vi "Main_04B.vi"() -> ()   [LabVIEW 2025]
uses:
  Utility/Universal Utility/TypeDefs_Utility/ENUM_8 Directions U-D-L-R.ctl
  Utility/Universal Utility/TypeDefs_Utility/Cluster_Row-Column.ctl
  b43e3300-6143-4e08-a70a-80936fe279ff.vi
  9e3f57c0-2ef8-4495-8287-c6a42a5fb955.vi
  <vilib>/Utility/error.llb/Trim Whitespace.vi
  <vilib>/Utility/error.llb/Trim Whitespace One-Sided.vi
  Utility/Universal Utility/TypeDefs_Utility/ENUM_4 Directions U-D-L-R.ctl
panel:
  out "sum":u32
  out "Array":bool[][](array[boolean])
  out "MATCH":bool
  in  "Select Data":enum32{"Example", "Puzzle"}(tab)
  in  "EX Target":u32=43
  in  "Example":string="..@@.@@@@.\n@@@.@.@.@@\n@@@@@.@.@@\n@.@@@@..@.\n@@.@@@@.@@\n.@@@@@@@.@\n.@.@.@.@@@\n@.@@@.@@@@\n.@@@@@@@@.\n@.@.@@@.@."
  in  "Puzzle":string="@@..@.@.@..@@.@@@@@.@@@@@@..@@.@@.@@..@@@.@@@.@.@@@@.@@@.@@@.@..@.@@@@..@@@.@@..@@@.@@@..@@@@..@.@@.@@@.@..@.@@@.@@@..@@@.@.@@@@@.@.@.@@@@@@\n@.@@@@@@....@..@@@.@..@.@.@@.@@.@@..@@@..@.@@..@..@@@.@@@.@..@.@.@@..@@.@..@@.@@@..@.@@.@.@..@@...@@@@@@@@.@@@.@@@.@@.@@@@@@@..@..@@@.@.@@.@\n.@.@@@@.@@.@@.@.@.@@.@..@@.@@..@@@@@@@@@@@@...@@.@...@@@@.@.@@.@@@.@.@@..@@.@@.@@.@@..@...@@@@.@@@@@@@@@@@.@@@....@@@@@.@.@...@@.@@@@@@@.@@@\n@@@..@@@@.@@@@@@@@.@@@@@.@@.@....@.@..@.@@@@@@@...@@@@@@@@.@@...@.@@.@@@@@@.@....@@.@@@.@.@@..@@@.@.@@@..@.@.@@@.@.@@@@@@@@...@.@@@@@@.@..@@\n@.@@@@@.@@.@.@.@.@..@@@@.@..@...@.@@@.@.@@@@.@@.@@@@@@.@@@@@..@@..@.@.@@.@.....@@@.@@@.@..@@@.@@.@..@@@@.@.@@@@..@@@@@@.@@@.@@.@@..@@.@.@@@@\n@@.@@@@@.@@@.@@@@@.@@.@.@@@@.@@...@.@@@..@@.@@.@@@..@@@...@@.@@@@..@@@@@@@...@.@@@@@@....@..@@@@@.@...@.@.@@.@...@@@@.@.@@@.@@.@.@@@@.@.@@@@\n...@.@@.@@.@.@.@@@@...@@@@@@@@@.@.@@@.@@.@@@.@@.@@@@.@@@@@@@@@.@@..@..@.@@@@@@@@@@@@...@.@.@@@.@.@.@.@@@.@..@@@@@@@@@@@.@@.@...@@@@@@@@.@@@@\n..@@@.@.@.@@@@@...@@..@@..@@.@...@@@.@.@.@.@.@@.@.@@@.@@.@.@@@@.@.@@@@@@@.@@.@.@@@@@@.@.@@@@@@@@@@@.@.@@@@@.@@@@@@@@@.@...@@@.@@@@.@..@@@@..\n.@@@@.@@@.@.@@@.@@@..@@..@@@@@@.@..@.@@.@.@@@@@..@@@@@@@@.@.@@@.@@@@@.@.@@@@...@@.@@@.@.@@@@@@.@@.@.@@@@.@.@@@.@.@@@@@.@@@@...@@@@@@@@@@.@..\n@.@....@@.@..@@@.@.@..@@@@.@.@@.@..@@.@.......@.@@@@@@@.@@@@@@@@.@@@.@.@@.@@@@.@..@.@@@@@@.@@@@....@@.@@@@.@..@@@.@@.@.@@@@@@@@.@@@@.@.@@..@\n@@@@@.@@.@.@.@@.@..@@@.@.@@@@.@@@.@.@.@@@.@.@@@.@@@@@..@@@@@@..@@@@@@@@@@@@@@.@@@@.@@@@...@.@@@@..@@@@@@@.@@@@.@@.@@@@@@.@@@.@.....@@@@@@.@.\n@.@@...@@@.@@..@@@@..@@.@@.@...@@@@@...@@@@.@@@.@@.@..@@@@..@.@@@@..@@@.@..@@@@..@.@@.@.@.@@....@.@@..@@.@@..@@@@...@@.@..@@@@@@@...@@@..@.@\n...@.@...@@@..@..@.@@@@.@.@....@@@@@@.@..@@@@@.@@@@@@@@@@.@@@@@@@@.@@..@@@@@@@@@@@@@@.@.@...@@....@@.@@.@@@.@@@@@@.@.@..@@@@@@.@.@.@@..@@@@.\n@@@@.@@@@.@.@@.@.@..@@@..@@@.@@@@@..@@@@@@.@...@.@@@.@.@..@@@@@@.@@.@@@.@@..@@@@@@@..@@@@@@@@..@@..@@@@@..@.@.@@@.@@..@.@.@@@@@@@.@.@@@.@@@.\n@@@@@@@@.@@@@@@@.@@@.@.@.@@.@..@@@@@@@.@@..@@..@.@..@.@@@@@@..@.@.@@.@.@@@.@.@@@@..@@@@@@@@....@.@.@@@@@@@@@.@@@..@@@@@@..@@@@...@@@...@.@.@\n..@@@..@.@@.@.@@...@@@..@.@@@...@..@@.@@@@@..@@@@.@@@@.@@@.@@.@@.@@@@@@@..@.@..@.@.@@@..@@@@@...@@..@....@......@.@.@.@.@@@.@.@@@@@@@.@@.@@.\n.@@.@@@@@.@..@@@@@@.@....@@@.......@..@@@.@@@...@..@@..@@@@..@.@@@@.@@.@@..@@.@.@@@@.@@.@@.@@@@@...@@@@.@@@..@.@.@@@.@.@@.@@@..@@@..@@@@@..@\n@.@.@..@.@.@.@@.@@@@@@@@@@@@.@@@@.@@..@.@.@@@..@@@@.@@@@@...@.@@.@@@@@@@...@@..@@@@..@@....@.@@@.@.@@@@@.@@@@@@@..@@@@@@@@@.@@@@..@@@.@....@\n@@..@@.@@.@.@..@@...@.@.@.@@....@@@@@@.@.@@@@@@.@..@@@@@@.@@@@..@.@.@.@.@.@@.@@...@@@.@.@@.@@.@@@@@@@.@..@@.@.@.@@..@.@@@@@@@@.@@@@..@@...@.\n.@@..@@@@@@@.@.@@@@.@@@@@@@@.@.@@@@@@@@@.@@@@@.@@@@..@@@@..@.@@@@.@.....@.@@.@@.@@@@@..@@@@@.@@@@@.@@@.@@.@@@..@@@..@@@@.@@.@@@@@@@@@@@@.@@@\n.@..@@@@@@@@@@@.@@.@@.@..@..@@@...@@..@@@.@@.@.@@.@.@..@@.@@.@@@@@.@@@.@.@@@@.@@@@@.@...@@.@@.@.@@..@@@.@@@@@.@@@@@.@....@@@@@@@@.@@.@@@@@@@\n@..@@..@@@@.@@.@.@.@.@.@@@@..@@.@..@.@@@@@@@.@@..@@@@@.@@@.@@@.@.@@.@@.@@@.@@@@@@@@@@@@@.@@@@@@.@@@@@@@...@@@@@@@.@@@@.@.@.@@@.@@@.@..@@@..@\n@@@@@@@@.@.@@..@.....@.@@@...@.@@..@@@..@..@..@@@.@@@@@@@@.....@..@@.@.@.@.@@@@.@@.@@.@@@@@@.@.@.@@.@@@@@.@.@@@...@@.@@@@@@@...@.@@.@@@..@.@\n.@@@@@@..@.@@...@@@@@@@@@@@.@@@@@..@...@.@.....@@@.@.@@@.@@...@.@.@.@@@@@@.@@@@@@.@@@@@...@@@@.@..@@.@@@.@@.@.@@@..@@@@@@@@.@@@.@@..@.@.@.@@\n@.@@.@@@.@.@.@.@@@@@@@@.@@@@..@.@@@@@.@@.@@....@..@@.@..@@@....@@..@@.@@@@@@@@@....@@.@@@.@@..@...@@@@@@@.@@@@@.@@@.@@@@@@@@@@...@@.@.@@@@@@\n@@@@@@@@@...@.@.@@@.@@.@@.@.@..@..@..@..@.@.@@@.@@@@@@@@@...@@@@@@@@@@.@@@.@@.@@...@@@@@@@.@.@@.@@@@@.@.@@..@..@....@.@@@.@...@..@..@@.@@@@@\n@@@@@@@@...@@@.@@@....@@@.@..@@@@.@@@@@..@@@...@@.@.@@@.@@.@.@@.@.@@@@.@@.@@@@@@@@@@@@..@@....@@.@@@@@.@@@@@....@@@....@@@@@.@.@@.@@..@@@@@@\n.@@@@.@@@@....@..@.@@@@@.@@@@@@..@..@@.@@@@.@@@..@@@...@.@@@.@.@@@@@@@..@..@...@@@.@@@.@@@..@@@@@...@...@..@@@@@.@@..@@...@@@.@@@@@.@@@...@@\n@..@@@...@@@.@.@@@@.@@@@@@.@@@@.@@.@@@@@@@..@@@..@@@@.@@@@..@@@..@.@@@...@@.@@@@..@@@@@@@@.@@@.@@...@@...@.@..@.@.@@.@.@@@@.@@.@..@@..@..@@.\n@@@@@@@..@@..@@.....@@..@@@..@@@@@..@@@@@.@@@@@.@..@@@@..@.@@@@...@..@@@.@.@@@..@@@..@@@@@..@@@@.@.@.@@.@@@@@@...@@@@@@@@@@..@@.@.@@.....@@@\n.@@@@......@@@.@@..@@@.@..@.@@@@@@.@.@..@@.@@@.@@@@....@@@@.@@.@@@@@@@.@.@@@..@@@.@@@@@@..@@@.@@@@.@@@@@.@@@@@@@.@@.@@@@@@.@@@@@@@@@.@..@@@@\n....@@@@@.@.@@@@@@@@@.......@.@@@@@@..@@.@@@@.@@@..@@@.@..@@@.@.@@.@@@.@@..@@@.@@@@@@@.@.@@@@@@...@@.@..@.@@.@.@@.@@@@@.@@@@@.@..@...@@@.@@@\n@@@@@@@@@@@@.@@.@@@.@@.@@.@@@..@@@@@.@@@.@..@.@.@@.@@.@@@@@..@@.@@..@....@..@...@@@@@..@..@.@.@@..@...@@@@..@.@@@@@@@@.@@@@@@@@@.@..@.@@@@@.\n@.@..@@@@..@@.@@.@.@@@@@..@@@@@@@....@@.@@..@@.@@@@...@@@@.@@@@@@@@@@.@.@@.@..@.@@@@@@@@.@@@..@@..@..@@@..@@@@....@@@@@@.@@..@@@@@@@@@@@@@@.\n.@@.@.@.@@@@@@.@@@.@@@@.@..@.@@.@@@@..@@@@@@.@@@.....@.@.@....@.@@@@@.@@@@.@@@@@@@@@@.@@@.@@@@@@@..@@..@@.@...@.@@@.@.@.@@.@.@@@@@@..@@@@.@@\n@.@@.@@@@@@@@@.@.@@.@@@@@@@.@@....@@.@@.@@@@@.@@@@.@...@@.@@@@.@@@@@.@..@@@@@@@.@@..@@@@@..@@.@...@@.@@.@@@@.@@@@..@..@@@@@.@@@.@@.@@@@@...@\n@.@@@.@.@..@.@@.@.....@.@.@@@@@@@@@.@@@@@@@@@@.@..@.@@.@@...@@@.@.@@.@.@.@@.@@@..@@@@@@.@@@@@@@@@.@....@.@@@@@@.@@@@@.@@.@.@@@@@@@.@@@@@@@.@\n@.@...@@@...@@.@@..@@..@.@.@@..@.@.@..@..@@@@@@@..@@@@@@@@@@.@@.@@@.@@@@..@..@.@@..@@@.@.@.@@@.@.@.@@@@@@....@.@@@@@@@@@.@@@@@@..@@@.@@@.@@@\n.@@@@.@@@.@.@.@@..@@@.@@@@..@@@.@@.@@@..@@@.@@..@.@@@@@@..@@@@@.@@@.@@..@.@.@@@@...@@.@...@.@@@.@@@@.@@@.@..@@@@..@@@..@@.@@.@.@@.@.@.@@.@@@\n..@@@@..@@@..@.@@@@@.@..@.@@.@...@@@@@@@@..@.@@@@@@...@@@@.@.@@@....@...@@.@..@@@@@.@.@.@.@@.@@@@@.@@@@@..@@@@@@@..@@.@@.@@..@...@@@@@@@.@.@\n.@@@@.@@@@.@@@@@..@..@@..@.@.@@....@@@@.@...@@@@@@@@..@.@..@.@@@@@@@@@@@.@.@@..@.@@.@.@@@@@@.@@@.@@@.@@@..@@..@@..@.@@...@@.@..@..@.@@@.@.@@\n.@@@@@@@@@@@@.@@@.@@...@..@..@..@.@.@@@.@..@.@@...@@.@@..@@@@@@..@@@@@@@.@.@@@@@.@@.@...@@.@@.@@@@@@.@@@.@.@@@@..@...@@@@...@@.@@@@@@@@.@@.@\n.@@@@.@..@..@.@@@@@.@.@@@@.@.@.@.@..@.@@@@..@@@..@@..@..@@@@@.@.@@@@...@..@....@..@@.@...@@.@.@@@.@@@@.@@@.@@@@@....@@@@.@@@.@..@@@@@@@..@.@\n@@@@@@@@.@@@...@@..@.@.@.@@.@@.@@..@@@..@@.@@@@@@.@@.@@...@.@@@@..@@@@@..@@..@.@@@@@@@@@..@@...@@.@@@.@@@@@@@.@@..@@.@@@@.@...@.@.@..@@.@.@@\n@.@@@.@.@@@@@@@@@@@..@@...@.@@@..@@@@@..@.@@@..@.@@@@.@@@@@@@@@.@.@@@.@@@@@@@..@.@@...@@@..@@.@.@@.....@@@.@@.@..@@.@..@@@.@.@.@.@@@.@@.@@@@\n@.@.@....@@@.@@..@@@.@@@@@@@.@.@@.@.@@@@@@@.@@.@@@@@.@.@@....@.@@@..@@@@@.@@@@.@.@@@.....@@@@@@@@@@..@..@@@@@@..@.@@@@@@@.@.@@.@@@.@@@@.@.@@\n.@@@@.@@@.@..@@@.@@@.@..@@.@@.@.@@.@@@.@.@@@@@.@@.@..@.@.@@@@.@@@.@@.@@@..@.@.@@@..@@@@@@@@@@@.@@@@@@@@@.@@@@@@..@@@...@@@.@@.@.@@@@@@.@@@@@\n@@.@.@@@@@@@@@..@@...@@@@..@@@.@@.@.@.@@....@@..@@.@@..@@@.@@.@..@@.@@@@.@@@@@@@@.@@@@@@@@@..@.....@@@@....@@@@@...@...@..@@@@@.@@.@....@.@@\n.@@.@@...@@@@@@.@@.@@@@.@.@@@@.@@.@..@@@@.@...@@@@.@.@....@.@@@@@@@@@.@@..@@.@.@@@@@@.@.@@.@.@@@@@@....@.@@@@@.@.@.@.@@@@..@@@@.@.@..@..@@@@\n.@@@@@.@@@.@.@@...@@..@@@..@@...@@@@..@...@.@...@@.@.@@@@...@@@..@@@@@@@@@.@@.@..@.@.@@.@@@.@@@..@@@@...@@@@@@@..@.@@@@@@.@@.@.@@@@.@...@@.@\n@@..@.@.@@.@.@@.@.@@@..@@...@@@@@@@@@@.@.@@@@@@.@.@.@@..@@@..@...@@@@..@......@.@.@..@.@.@.@.@@@@.....@.@.@.@@.@@.@.@@@@@@.@@@@@..@.@.@..@@@\n.@@@@@@@@@@.@@@@..@.@.@.@@@@@@@@.@@@.@@.@@..@@..@@@.@@..@.@.@.@@@..@.@.@@@.@..@@@.@@.@.@..@@@...@.@@@@...@@@.@.@@.....@@...@.@@.@@@@@.@@@@@.\n.@@@..@@@@@@@.@@@.@@@@..@@@..@..@@@..@@@..@@.@@.@@@@@@@.@.@@@.@.....@@@@@.@@.@@..@@@@.@@....@@@..@@@@.@@@@@@.@@.@..@@@.@..@@..@..@@.@@@.@@..\n@@@@@@..@.@@@@@.@@@@.@..@.@@@@@..@@@@..@..@@@@@.@@@@@@@.@..@@..@@@@@@@@..@@@@.@.@@.@@...@.......@@.@..@@@@.@..@@@@...@.@@@.@......@@...@@@..\n@.@.@.@....@.@.@@.@@@@@@@.@..@.@..@@.@.@.@@@@@@..@...@...@.@.@.@.@@@@@@@@@..@@@.@@@@@@@@@.@..@@@@@@.@@.@@@@@@.@@.@@...@@@@@@.@@@.@@.@..@..@@\n.@@@.@@@@@@@@.@@@.@..@@.@..@..@@.@@@..@@@@@@.@@@@..@@....@@@@.@.@@.@@.@@@..@@@@@@@....@..@@.@@@@@..@..@...@@.@@@@@.@@.@@@@.@@@@@@.@..@.@@@.@\n@..@...@@@@..@@..@@..@@@.@.@@@@.@..@@@.@.@.@@@@@.@@...@..@@...@....@.@.@@@@@.@@@.@@..@@.@@@.@.@@..@@@@..@@@@@@@@@.@@@@@.@@.@@.@.@@.@.@.@@@.@\n@.@.@@@.@..@.@.@.@.@@@@@@@.@.@@.@..@@@.@@@@@@@...@@@.@@@.@@@@.@@@....@@@@@@@.@@.@.@@...@..@@.@..@.@@.@.@@@@..@@@.@@@@@@..@@@..@.@@@@@@@@@@.@\n.@@.@@@@..@..@@.@.@.@@.@@@@..@@.@....@@@@.@@@.@@@.@@@@@@@@.@@.@@@.@@@@.@@@@@@@@@.@@@@..@@.@..@@@.@.@@@@@@@@@@@.@@.@.@.@...@@@@@.@@.@...@@@@@\n.@..@@...@@.@@@@@@@@@@.@@@.@@.@@@@@@@.@@.@@@@.@@..@@.@.@@.@@@.@@@@.@.@@@@..@...@.@...@@@.@@@@@..@@@@@@@..@.@@@.@.@.@.@.@@.@@@@..@.@..@.@.@@.\n.@..@...@.@@.@..@@@@@@..@.@@@@@@...@@..@@.@@@@.@....@.@@@..@@@@..@@.@.@..@.@@.@.@.@@@.@..@.@@@@@@.@@@.@@.@.@..@@.@@.@.@@@.@.@.@.@@@.@@@.@@..\n.@@@.@.@..@..@@@..@@@.@@.@.@@@.@@@.@@@.@@@..@@@@@@..@@@@@@@.@@@@.@.@...@@@@@@@.@@@@...@..@@@@.@.@@@......@@@.......@@.@..@@@@@..@.@.@@@...@@\n.@@@@@@.@@@.@@@@@@@.@@.@@.@@@@@..@.@.@.@..@@.@.@.@@@.@.@@@.@@@.@@.@@..@@@..@@@@...@@..@.@.@@@..@@..@.@@@.@..@.@@@@@@@@@...@@@@.@@@@@@@.@.@.@\n@.@.@@.@@@....@@@@@@@.@@@...@@@..@.@@@@@@@@@@@@.@.@@@@@.@@@.@@.....@.@@@....@.@@....@@@@@@@.@@@@@.@@@.@.@.@@.@@@@@@@@..@.@.....@@@@@..@@@@.@\n@....@...@.@.@..@@@@@......@.@...@.@.@..@@.@@@@@@..@@@@.@.@.@.@.@.@...@@@@.@@@.@...@...@@@...@@@@@@@@@@@..@@@..@.@@@@@@.@@@@@....@@@.@@.@..@\n@@@@.@..@@@.@@@..@@.@@@@@@.@.@.@.@@@@@@@.@.@@.@@@.@@...@@.@.@.@@..@@@.@@@@@.@@.@.@@@@@.@@@@@@.@@.@@@@@.@.@@.@@....@@....@....@@@@.@@.@@@..@@\n@.@@@@@@@@@..@@@@@..@.@@.@..@@@.@@@@@@@@..@@@@@..@@@.@.....@@@..@.@@@@@@..@@..@@@.@.@..@.@@.@@@@@@.@.@@.@@@.@@.@@.@..@.@.@@@@..@.@@@@..@.@.@\n@@@@@.@.@.@@...@@...@@@@@@@@.@..@..@@@@..@@@..@.@@.@.@@@.@.@@@...@.@@@..@@@@@@@@@....@@@@@.@@@.@@..@@...@@@.@.....@@..@@@@@@@@@..@@@@@.@@@@@\n@@@..@@@.@@@@@@@@@@@@..@..@.@@.@@@@@@@@@@@@@.@@@@@@.@..@.@@@@@@@.@@@@@.@@@@@@@...@@@@@...@@.@.@@@@..@@@@@@.@@@@@..@@@@@@.@...@..@@@.@@.@.@@.\n.@@..@@@@@.@@.@@@@@@.@@@.@@.@.@@@@.@@..@@@....@@@@@@@.@@....@@@@@@.@@.@@...@..@@@@@@..@.@.@@@@@@@@@@.@@@@.@@@@.@.@@@@...@.@.@@.@.@@.@.@@@@..\n@.@@.@@.@@@@@@@@@.@@@@@@@.@@@..@..@.@...@..@..@.@....@@.@@.@@@@.@.@@.@@.@@.@.@@@@@@@@@@@.@.@@@..@@@..@@@.@@@@@@@@.@.@@@@@@@.@@.@..@@@@@@@@@@\n..@@..@.@@@@@.@@@.@@@.@.@@@@.@.@@@@@@@@@@@@@.@@@@...@@@@@@@@@@.@.@@.@...@@@@@..@@.@@@@..@@@...@..@@@.@@@.@@@..@@@@.@.@@.@@@.@.@.@.@@@.@@.@..\n@@..@@@@@...@@@.@@@@.@...@@@@@@@.@@@.@...@@@@@@@..@..@@@@@.@.@@.@.@@.@.@.@@@@@@...@.@....@@@..@.@@@@@@@@@@@@.@..@@@@@@@@@.@@.@@@@@..@@@@.@@.\n@.@@.@@..@...@@@@@@..@.@@...@@.@@@@@@.@.@...@@.@@@.@.@@@@@.@@@@@.@.@@@.@.@@@@@@@@@.@@@.@.@@@@@@@@@@@@.@.@@@.@@.....@.@@@@@@@@@@@@@@@..@...@@\n@.@.@.@.@.@@...@@@@@@.....@.@.@..@..@@@@@@@..@@@@@@....@@.@..@@..@.@@..@@@.@@.@@.@@@@@.@....@@@@....@.@@@...@..@...@@.@@@@@@@@@@.@@...@@@@.@\n@@@.@@@...@@@.@@@@@@@@.@.@@...@@@@..@..@@@@@..@@@@@@@@@....@@@@@.@@@....@.@.@.@.@@.@@@@..@@@.@@..@.@.@@@@@@@@@@@@@@@@.@.@.@@@@@....@..@@.@@@\n...@@@.@@.@@.@@.@@...@.@.@...@@.@@.@@.@..@@@@.@@.@@@@.@@.@@..@@@@...@@@@@.@..@.@@@@@@..@@..@@@.@.@.@@..@@@@@@..@@..@.@@@@@@@@.@...@@.@@.@@.@\n@@@@..@@.@@..@.@@@@@.@.@@@@.@@..@..@@.@.@@@@..@@@@@@@@@@@@@.@.@@@@.@.@@@@@@.@...@@@@.@.@@...@.@@@@.@@@..@@@..@.@@@@@..@.@@.@@.@@@@@@@@.@@@@.\n@@@..@@..@@@@@.@@.@..@@@.@..@.@@.@@..@.@.@@.@....@@@...@@@.@@@..@.@.@.@@@.@.@.@....@@....@@@@@.@@@@@@@.....@@..@.@@@.@@@@....@@..@@@.@@.@.@.\n@@.@..@@@@@@@.@.@@.@@@.@@@.@@.@@@@@@@@@@.@@@..@.@@@@..@@.@@.@.@.@@@.@.@@@@@@......@@@..@@@.@.@@.@@@@..@@.@@.@.@@..@.....@@@@@.@.@@.@.@.@.@.@\n@@@.@@@@..@.@@.@@@.@.@@@.@....@.@.@@..@..@@.@@@@@@.@@.@@@@.@@@@@@@@@@@@@..@.@.@@..@..@@.@@@@.@@.@@.@@..@@@@@@.@@@@@.@@.@@@.@@.@...@@.@@.@.@@\n@.@@@@@@@..@.@@@.@.@@@.@.@@@@@..@@@@@...@@@@.@@..@@.@.@...@@@@@@@@@@@.@@@@@@...@@@@@.@@@@@..@@@.@@.@..@.@@@@.@@.@@@.@@@.@@@.@.@@@@@@@@@..@@.\n@.@@.@..@@.@@@@@.@@.@@@.@..@..@@@.@.@.@@@@@.@@..@.@@....@@@@@.@..@@.@@.@@.@@.@@.@.@@.@@@.@@@.@@.@.@@@.@@@@@@@..@@@.@.@@.@.@@.@@@.@@...@.@@@@\n@@......@@@@@.@.@.@.@@@@..@@.@@@@@@@@@.@@@@.@@@.@@@.....@@@@@@@@..@@@@.@@...@@@@@@@@..@.....@.@@@..@.@@@@@@@@@.....@@@@@@@@.....@@.@@..@@.@.\n@@@...@@.@.@.@@.@@.@..@.@@.@@@@@..@..@.@@@@@@@.@@.@@@..@..@.@@@@.@@.@@@@@@@@@@@.@..@@@@.@..@@@@@.@.@@@@@@@@@..@@.@@@@...@@@@@@@.@@..@@.@@@@@\n.@.@@@.@@@@.@@.@@@@@...@@..@@@@@@@@@.@.@@..@.@@.@@@.@@@@@@.@@@@...@@.@@@..@...@@.@@@@.@....@@@.@....@....@@@@@@.@@@..@@.@@..@@...@@@..@.@@@.\n.@....@.@@@@@@@@@@...@@@@.@.@.@.@@@.@@@@@@@@@.@@.@@@..@.@.@@@@.@...@@@@..@.@@@@..@@.@@@@.@@@@@@.@@.@.@@.@..@@@@@@@@@@@@@@@@.@@@@@@.@.@.@.@..\n..@@@.@..@@..@@@@@@@..@@@.@@@@..@@..@@@@.@@@@..@@@.@@@.@@@@..@@..@.@.@.@@@@@@@...@@.@@@@@@.@@.@@@.@@@.@@@@@@@@.@.@@@@@@@@@.@.@....@@.@@@@@@.\n@.@@@.@@@@@.@@@@@.@@@...@.@@.@@@@@@.@..@.@@@@@@.@@.@@@@@@.@@@@@.@@@@@@...@@..@@@@@..@.@@@.@.@@.@.@.@@.@@@@.@.@..@@@.@.@@@...@@@..@@.@@@@@..@\n@@@.@@@.@@..@..@@@....@.@@@..@....@.@.@@@.@....@@@..@@.@@@@.@.@@...@..@.@@@.@@@@@@@@@..@.@@...@@@.@@@@@...@@....@@@@@@.@....@@@.@@.@@..@@@@@\n@.@..@...@@..@.@@@..@@@@@@.@..@@@..@@@@@.@@@@@@@.@..@@@@...@@.@@@@.@@@@@.@.....@@@@@.@@@@@.....@@.@..@@.@@@@@.@@.@@@@@.@@.@@.@@.@.@@..@.@.@.\n@..@@@@@@.@@...@.@..@@@@.@@@.@@@@@@@@.@..@@@@...@@@@@@@.@.@@.@@@@..@....@.@....@...@@.@@.@.@.@.@.@@.@@.@@.@@@..@@@@.@@@@.@@@.@.@@...@..@@...\n@@@@@@.@@@@@.....@@@@@@@@@@@..@.@@@@@@@@..@...@.@@.@@@@.@@@.@@@.@.....@.@@@.@@..@@@@...@@..@.@@@@.@@.@@@@..@@.@..@@@@@@@.....@@.@...@@..@.@.\n@@@.@@@@..@@.@.@@@@..@.@@.@@..@@@..@@.@@.@@...@@@@@..@..@@@@.@@.@@@@@.@@@..@@.@@@@..@.@.@...@@.@@@@@@..@@@@@@@..@@@@@@@.@.@.@.@.@...@@@.@@.@\n@@@@.@..@@.@.@.@@@.@..@@.@@@@@@@..@@@@@@@@@@@.@@@@@@.@@.@.@@.@@..@@@.@@@@@.@@.@..@@@.@@@@.@@@....@@@@@@@.@....@.@@@@@@@.@@@@.@@@...@.@@.@@@@\n@@.@.@@...@@@.@@..@@.@@@@.@@.@@.@..@.@..@@@@@@..@...@@..@@@.@.@@@@.@@.@@@.@.@@.@.@@@@@...@.@.@@@..@@@@.@@@@@.@...@@@.@@@@.@@.@...@.@@@.@@@.@\n@.@.@..@@@@..@@.@.@..@@@@@.@@@.@....@@.@..@@.@.@..@@..@....@@@.@@@..@@.@@@@@@.@.@.@@@@@.@@..@.@@.@@@..@@@.@@.@@@@..@@@@@@@@@.@@@@@@.@@@@.@.@\n.@.@@.@@@.@..@@..@@..@@@.@.@@.@@.@@.@....@@.@@.@.@@@@@.@@@.@.@....@.@@@.@@@@@@@@@@.@@@..@@@@....@@.@@...@.@@...@.@@....@...@.@@.@.@@..@.@@@@\n.@@@@@@.@@@@@@@..@@@@@@@@@@..@..@@@@@@@@@@....@.@@@@@@.@@@@@@@@@.@@..@.@...@......@.@@@@@.@.@.@@.@@....@@..@@@..@@.@@.@..@@@.@@...@@@@@@@@@.\n@@@.@@@@@@.@...@.@@...@..@@@@.@@@@@..@.@@.@@@@@@@....@@@.@.@@.@..@.@.@@.@.@@..@.@@@@.@....@...@@@.@@@@.@@@@@@@@.@...@@@@@@@@@@.@@@..@.@..@@@\n@@@@.@@..@..@@@@.@.@@@..@@.@@@.@@.@@.@@@..@@@@.@@@@@@.@@..@.@@@.@.@@...@..@@@...@.@@.@@.@.@@@@.@.@...@@@.@@@.@@.@.@@.@@.@@@@@@.@@@@.@@..@@@@\n.@.@.@@@@@@@@@.@...@..@@.@@@@@@@@@.@@@@.@@..@@.@@.@@@@.@@@@@@@..@@..@...@@.@@@@@@@@@.@@@@@@@@@@@@....@.@@@.@.@@@..@@..@@.@@.@@.@..@@.@.@@@@@\n.@@.@@@....@@...@@.@@@.@@...@@..@@.@@..@@@@...@@@@@..@@.@..@.@@@.@.@..@..@@@@.@@..@@......@.@@@@@@.@....@.@.....@@@.@@.@@@@..@@.@@@@..@@..@@\n..@.@@@@@.@@.@..@..@@.@@@@.@@@...@..@@@.@..@@@.@@@.@@...@@@@@@.@@.@.@@@@..@@@@@.@@@.@.@@@@@...@...@@@@.@@@@@.@@@@@@.@@@.@@@@@@..@....@.@....\n......@.@@@@@@@..@@@..@@@@@.@@@.@@@.@@.@.@.@@..@@@@.@.@@...@.@@@@.@@.@.@.@@@@@.@@@@@@@...@@.@@@@@..@@@.@@@.@.@@@@...@@@@@@.@@@.@@@@.@..@@@.@\n@.@@@@.@@.@@.@.@@.@@@@@@@@@@@@@@@@@@@@@@.@@@@.@.@.@@@@.@..@@@..@.@..@@@@@..@@@@@.@..@@.@@@@@@.@@@@@@.@@.@@@@@.@@@.@@@@.@.@@@@@@..@@.@@..@@@@\n.@@@@.@@@@@@@@.@@@@@.@..@.@..@..@@.@@@@@...@@@.@@@@@@.@@@@@@@@.@.@@@@..@@..@@@.@@@@@@.@.@@@@@@@.@@@.@..@.@@.@.@..@@@.@@@@@.@@@@@...@@@.@@.@.\n@...@@@@..@@.@@@.@@@.@@@@@.@@@....@@@@@@@@@@.@@..@.@.@.@.@@..@.@@@@@.@@.@.@@@@@.@@@.......@..@@......@@..@@.@@@.@@@@@@.@.@@@@@.@@@@.@@@@..@.\n.@@....@..@.@.@@@@@@@@@@@@..@@@@.@@@@@@@@@..@@.@.@@@@.@@.@@@@@@@.@@@..@.@.@@@@.@.@@@@@@@@.@@@@..@@@..@@@.@@@.@@@@......@@.@@..@@.@@@@.@...@.\n@@@@@@@@@@@@@@@@@@.@@.@...@@.@..@@.....@@@@@@..@@.@.@@..@..@@@...@@....@@@@@.@@@@.@@.@@@@.@..@@.@@.@@@.@@@......@...@...@@@@@@@@@@@.@@@@@.@@\n@@...@@@.@@.@.@.....@.@@@@@@@.@.@.@@@..@@@@@..@@.@@@@@@@@@@@@@@@.@@..@@@@...@@@.@@.@@.@@@@@.@..@@@.@@@@@..@@....@.....@@@..@@@@@@@@....@@@.@\n@@@@.@.@@@@@@@@..@..@.@@@@.@.@@..@@@@@@@.@@@@.@..@@@@@.@.@.@@@@@@..@.@.@...@@@@@@@@....@.......@...@@@@@@@.@.@..@@@@@..@@@@@@.@@@@@@.@@.@@@@\n@.@@@@@.@@@@..@..@.@@..@@..@@@..@@.@@...@@@.@.@@.@@@@@@@@@@..@@.@@@@@@.@@@..@@.@@@@@@@.@.@@..@.@..@@.@@@@.@@.@@@..@@.@@@.@..@@@@.@@@@.@.@@@@\n.@@@@@@@....@...@.@.@@...@@@@....@..@.@@@@.@.@@@@@.@@.@.@@@....@@.@@.@.@...@@.@...@.@....@@@.@@.@@@@.@@@.@.@.@.@@.@@.@@@@.@@@@@@.@@@@.@@@@@.\n@@@.@@@@.....@.@.@@@.@@....@@..@@.@@@@.@@.@@.@.@@.@@@@@@@@@@@@@@@..@..@@@@@@..@@@.@@.@..@...@@@.@@@@.@@@.@...@@@@@@@.@@@.@@.@@.@.@@@@@@@@.@@\n..@@@.@.@@.@@.@@.@@.@@...@@.@@..@.@.@.@..@@@@.@@..@@@@@@@@.@@@@@@@@.@.@.@@.@.@@..@@.@@@@@.@@@...@@@.@.@..@..@@@@@.@@..@@@@@@...@.@...@@@@@@.\n@@.@.@@..@@@@@@@.@.@@@@.@.@.@.@@@.@.@@@..@.@.@.@@.@@@@@@@@..@.@@.@....@.@@@@@@@@@@..@..@@@@@@@..@.@@@.@@@@@@@.@@..@.@@@@@@...@@@...@@@@@...@\n@@@@@...@@@@..@@@@@@@@@@.@@@.@@@@@@.@.@@.@@...@..@.@@@...@@@..@@.@.@@@@@@@@@@...@@.@@.@@@.@@@.....@@@@@.@@@@@@@@.@@@...@@.@@..@.@@@@@@@.@@@@\n...@@@@@.@.@.@.@..@@@@.@@@@@@@@@@...@.@.@@@...@@@..@@@@@.@@@@@@@@@@@@@.@@@@@@.@...@@@@.@@@@@.@.@@.@...@@.@@.@@@@@@@@@@@@@.@@..@.@@@@.@@@.@@@\n@@.@@..@@@@.@@..@@@.@@.@.@@@@.@@@.@@@..@@....@@@@..@@@...@@@.@@@.@.@@@.@@..@@@@@..@..@@..@@..@.@..@..@.@@@@.@.@.@@@@@@@.@@.@@@@@@..@@..@.@..\n@@@.@@.@@@.@@@.@..@.@@...@@.@@@.@..@.@@.@....@@@.@.@@@.@.@@.@@.@@.@@.@.@.@@.@..@.@.@@.@@.@@.@.@@@@@...@@@@..@@.@@..@.@@@@@@..@@@@.@@@@..@@..\n@@.@.@@@@@@@@@@..@@..@..@@@@@..@@@.@.@@@.@@@@.@@....@@.@.@@..@@.@@@@.@@.@@@@.@@.@@.@@@@.@...@@.@..@@@..@.@.@@.@@@@.@.@@@@.@.@@.@.@..@.@@.@.@\n@@@@@..@@.@...@@@@@.@@@.@@@@@@@.@@@.@@@@@@@@@@@.@@.....@..@..@.@@@@@@@@@.@@@.@@.@@..@.@........@..@.@@@@@@@@.@@.@.@.@@.@@@@.@....@@.@.@@@@.@\n@@@.@..@.@@.@@@@@..@@@@.@@..@@@@@@@@@@@.@@@@@@@..@@.@@.@@@@@@@@.@@@@@...@.@..@.@..@..@@@.@@.@@@.@@.@@.@....@@@@@@@@@.@@..@.@@@@...@.@@.@@@@.\n.@.@@...@@.@@.@.@@@@.@@..@@..@..@@.@@@.@@@@.@.@@.@.@@@@@@@..@@@.@@@@@@@@.@@.@@@..@..@@@@@.@@@.@.@@@@.@...@@@@@@@@@@.@@.@@.@@@.@@@@.@.@@..@..\n@..@.@..@@...@.@@@@..@@.@@@.@@@@@.@.@@@@..@@@@@.@@@@.@.@@.@@.@@@@.@@@..@@@@@..@..@@@@@@@.@...@@@@..@@@@@@@.@.@...@.....@@@@@..@.@.@@.@@@@@..\n.@.@@@@...@@@.@@@@@.@@@@@@.@@@@@@..@@..@@@@.@@@@@@@@@@@@@.@@@@@@..@@@@@.@@@@@@@@@.@...@@@@@@@.@.@@.@.@@@..@@@@@@@..@..@@@@@@@@..@@@...@@@.@.\n.@@@@..@@@@@@@@@@@@@@...@.......@.@.@@@@@@.@.@@@@@@@@@@@...@.@@@@@@.@.@@@@@.@.@@@@@.@.@@..@..@.@@@.@@..@@@@..@@@@@@.@@@@.@@@@..@@@.@..@..@@@\n...@@@.@..@@@@@.@@@@@@@.@.@.@....@@@@.@@@.@@@.@@@@@.@.@@@.@@@@@@@@.@@@@..@@.@@...@@@@@@@@@@@@@@@@.@@@@.@@@..@@@@.@@.@..@@...@@@.@@@@.@..@..@\n@..@.@@@@@@@..@@@@..@@@@..@.@@@@@@@@@@@.@@@@@@@@@@@@....@@.@@@@@@@@@@@@@@@@@.@@.@.@.@@.@.@.@@@@@@@@@@@@@@@...@@@@@.@@...@@@...@@..@@@@..@.@@\n@.@....@@@@@@@@@@@.@@@.@@.@@@@.@..@@@@@@.@@..@@@@@@...@.....@.@@...@@..@@...@@@@@@@@@@.@@@@@..@...@.@@.@@@.@@@@...@@@@@..@@@@..@@@@@.@@@@...\n@@..@@@@@@@@@@.@.@@@....@@@@@@.@@.@@@@@..@@@.@@..@.@.@@@@@@.@@@@@@.@@...@@@@@@@@@.@@@@@..@@@.@@@.@.@@@@@@@@@@.@..@.@@@@.@@@..@@@@.@@@..@..@@\n@@@....@..@@@@@@@@@@.@...@@.@@@@@@@@@@@@@..@@..@@..@@@..@.@@.@@@@.@@.@@@@.@@.@.@@@.@..@@@@@@@@.@.@@@.@@@@@@@@.@@.@@@.@@@.@.@.@@@@..@@@.@@.@.\n@@@@.@@@..@@@@@@@...@@@@@.@@@.@@@@@@@@@.@@.@.@@@.@@@.@.@.@@@@.@@@@@@.@@.@@....@@@@@@@@@.@@@.@@@.@@@..@@....@@@@.@.....@@@..@@@@@..@.@@.@@@@.\n@@.@@@@.@.@@.@@.@@@@@@@@@@@.@.@@.@.@@.@@@@...@@.@.@@@@@@.@.@@@@@@@..@.@@.@@@@...@@..@@@@@@@@@.@@@.@@.@@.@.@..@.@@@..@@.@@@.@...@.@@.@@..@@@.\n@@.@@@@@@@@@@@.@@@@.....@.@@@@.@@.@@@@@.@@@@...@@@.@.@@@@@@@@@..@@.@.@.....@@@@@@@@@@@@@@@@@..@.@@@.@@@@@.@@@.@.@@@@@.@.@.@@@@@@.@@@.@..@@.@\n@.@.@@@@@.@.@@...@@@@@@..@@.@@@@@@.@@..@@@@...@...@.@.@@@@@@@@@@@@@@...@@@..@.@@.@@.@.@@.@@...@@@@@..@@@...@.@@.@@@...@@@@.@@.@.@@..@.@@@@@.\n@@@.@@.@@@@..@@@@@@.@@....@.@.....@@.@.@@.@@.@@@@@...@..@@...@@.@@@@@.@...@@@@.@@.@..@@.@.....@@@@@@@@@.@.@@@...@.@.@.@.@@@...@@@@@@..@@@@@@\n@.@.@@@@@@@@@@.@.@@@..@..@.@.@..@.@@@@.@@@@@@.@@@@@@...@.@.@@@.@.@@@.@.@@..@@.@@@.@.@.@@.@..@@.@..@@@@@..@@..@@.@@@..@..@@@...@@@@.@..@..@@.\n.@@@@@@@..@@@.@@.@.@@@@.@.@@@@..@@..@@@..@.@@@.@@@@@@@.@@..@..@..@@@..@@@.@@@@.@@@.@@..@@@.@.@@@@.@@@@@...@.@@.@@.@@@@..@..@.@@...@.@@..@@.."
  in  "Puzzle Target":u32=8948
  out "Answer":u32
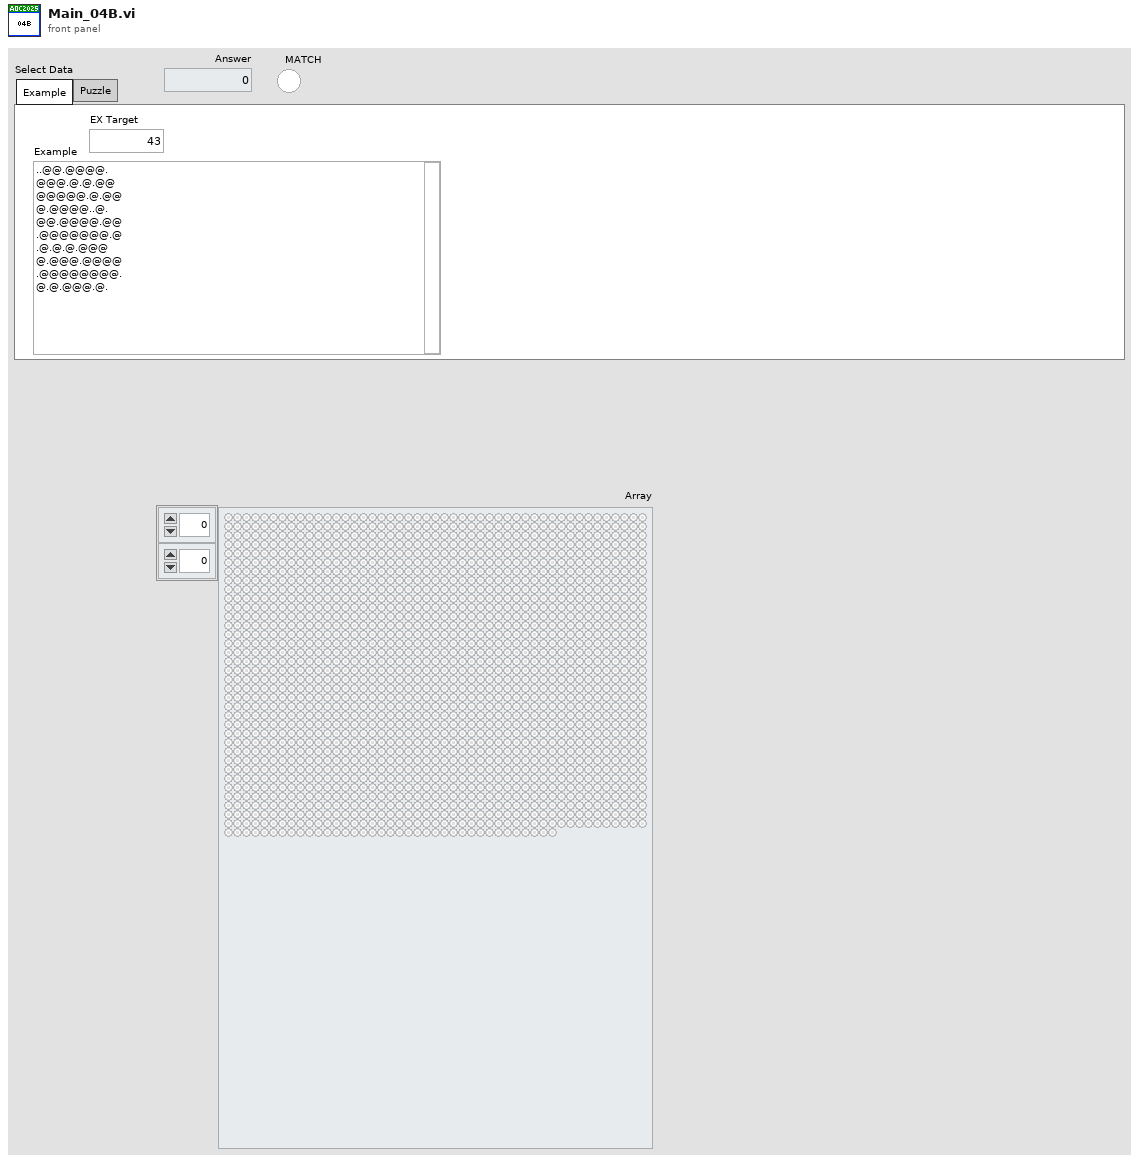
[diagram p1: front panel]
types:
  T1 = typedef "ENUM_4 Directions U-D-L-R.ctl" = enum16{"Up;-1,0", "Right;0,1", "Down;1,0", "Left;0,-1"}
  T2 = typedef "Cluster_Row-Column.ctl" = cluster{"R":i32, "C":i32}
  T3 = typedef "ENUM_8 Directions U-D-L-R.ctl" = enum16{"Up;-1,0", "Up-Right;-1,1", "Right;0,1", "Down-Right;1,1", "Down;1,0", "Down-Left;1,-1", "Left;0,-1", "Up-Left;-1,-1"}
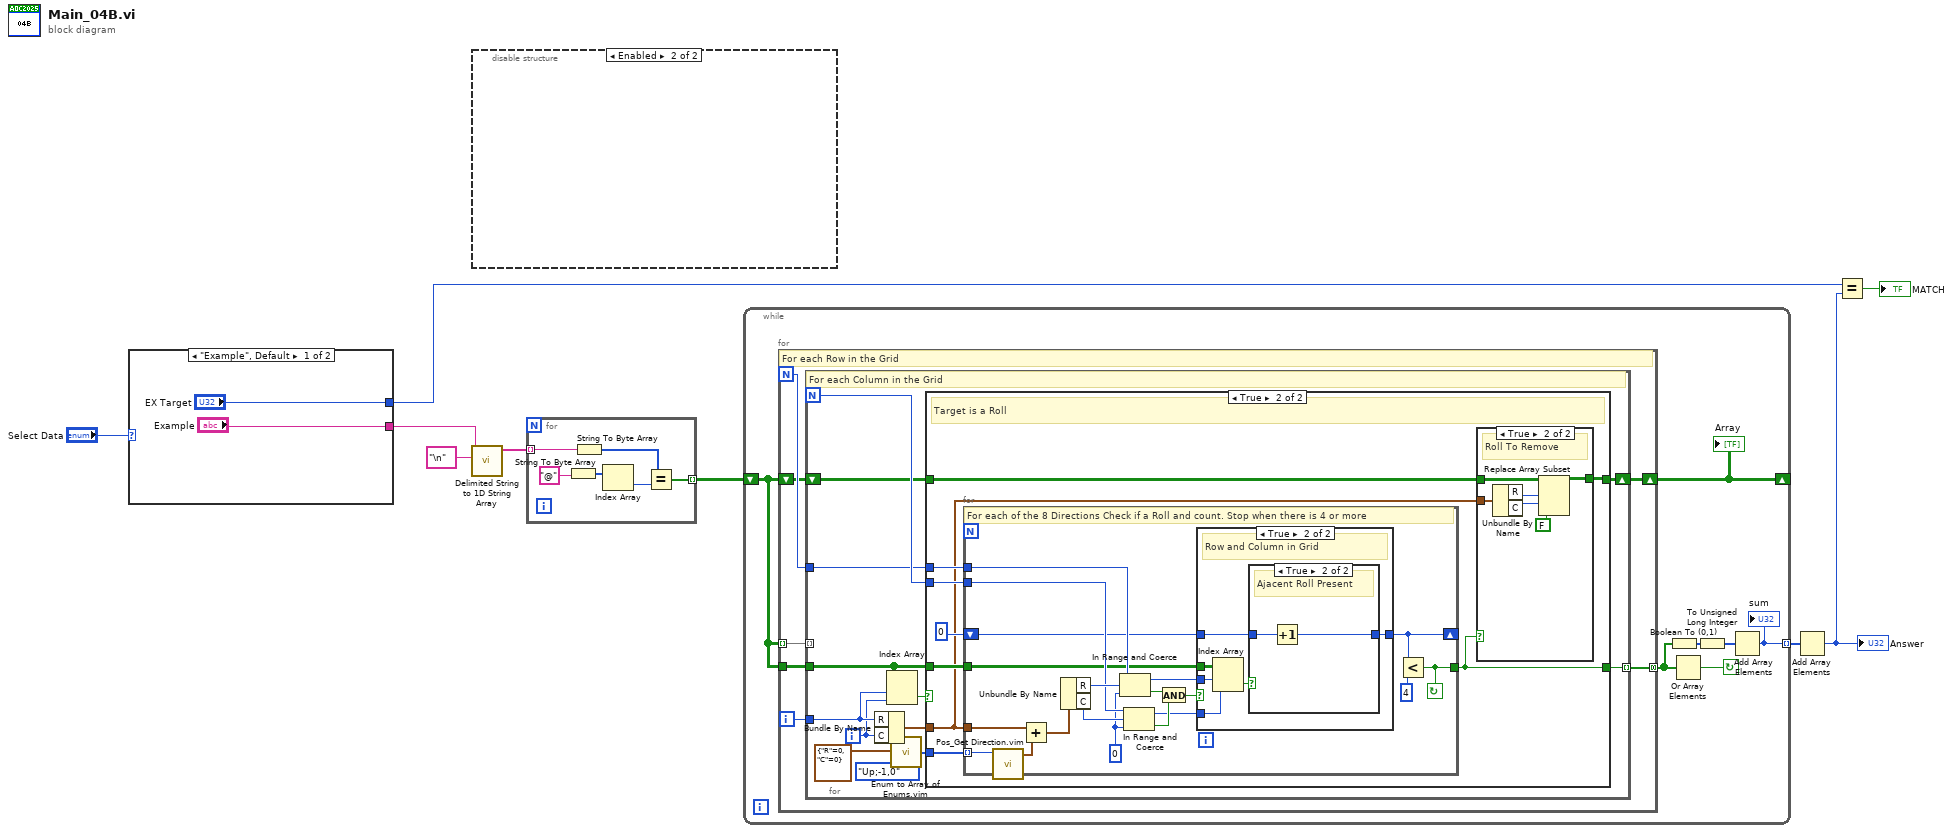
[diagram p0: block diagram]
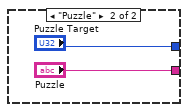
[diagram p2: hidden frame]
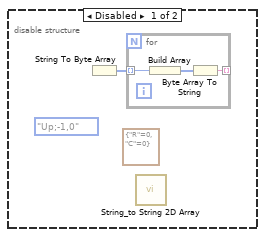
[diagram p3: hidden frame]
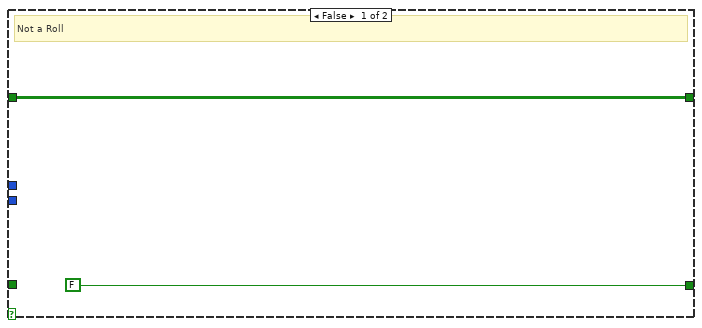
[diagram p4: hidden frame]
diagram:
  n1 = case shown="\"Example\", Default" "Select Data" {
    tunnel: ["Example" "Puzzle"] -> w7
    tunnel: ["EX Target" "Puzzle Target"] -> w4
    frame "Example", Default {
    }
    frame "Puzzle" {
    }
  }
  n2 = call <vilib>:"Delimited String to 1D String Array.vi"("delimiter"="\n" ("delimiter (Tab)"), "delimited string"=w7) -> ("string array"=w8:string[])  [unwired: 9 in]
  n3 = disable-structure shown="Enabled" {
    frame Disabled {
      (unwired) ENUM_4_Directions_U-D-L-R."Up;-1,0" ("Direction")
      (unwired) T2 {"R"=0, "C"=0} ("Position")
      n4 = String To Byte Array() -> (unsigned byte array=w14:u8[])  [unwired: 1 in]
      n5 = for {
        tunnel: w14 -> [w17] mode=indexing
        tunnel: [w15] -> _ mode=indexing
        n6 = Build Array(w17) -> (w16:u8[])
        n7 = Byte Array To String(unsigned byte array=w16) -> (string=w15:string)
      }
      n8 = call "String_to String 2D Array.vi"() -> ()  [unwired: 11 in, 1 out]
    }
    frame Enabled {
    }
  }
  n9 = for {
    tunnel: w8 -> [w19] mode=indexing
    tunnel: [w18] -> w3 mode=indexing
    n10 = String To Byte Array(string="@") -> (unsigned byte array=w21:u8[])
    n11 = String To Byte Array(string=w19) -> (unsigned byte array=w23:u8[])
    n12 = Index Array(array=w21) -> (element=w22:u8)  [unwired: 1 in]
    n13 = Equal?(x=w23, y=w22) -> (x = y?=w18:bool[])
  }
  n14 = while {
    shift-right: [w24] -> _
    shift-left: w3 -> [w30]
    tunnel: [w25] -> w2 mode=indexing
    stop <- w29 continue-if-true
    n15 = for {
      N -> [w35]
      tunnel: w30 -> [w37]
      tunnel: [w34] -> w28 mode=concatenating
      tunnel: w30 -> [w33] mode=indexing
      shift-right: [w31] -> w24
      shift-left: w30 -> [w32]
      i -> [w36]
      # "For each Row in the Grid"
      n16 = for {
        N -> [w47]
        tunnel: w37 -> [w44]
        tunnel: w36 -> [w43]
        tunnel: w35 -> [w46]
        tunnel: [w45] -> w34 mode=indexing
        tunnel: w33 -> [_] mode=indexing
        shift-right: [w38] -> w31
        shift-left: w32 -> [w40]
        i -> [w42]
        # "For each Column in the Grid"
        n17 = Bundle By Name(cluster=T2 {"R"=0, "C"=0} ("Position"), "R"=w43, "C"=w42) -> (w39:T2)
        n18 = Index Array(array=w44, index (row)=w43, index (col)=w42) -> (element=w41:bool)
        n19 = call "Enum to Array of Enums.vim"("enum"=ENUM_8_Directions_U-D-L-R."Up;-1,0" ("Direction 8")) -> ("array of enums"=w49:T3[])
        n20 = case shown="True" w41 {
          tunnel: w49 -> [_ w61]
          tunnel: w39 -> [_ w53]
          tunnel: w47 -> [_ w59]
          tunnel: w46 -> [_ w58]
          tunnel: [FALSE w54] -> w45
          tunnel: w44 -> [_ w57]
          tunnel: w40 -> [w51 w55]
          tunnel: [w51 w56] -> w38
          frame False {
            # "Not a Roll"
          }
          frame True {
            # "Target is a Roll"
            n21 = for {
              tunnel: w61 -> [w87] mode=indexing
              tunnel: w53 -> [w86]
              tunnel: w57 -> [w73]
              shift-right: [w71] -> _
              shift-left: 0 -> [w72]
              tunnel: w59 -> [w81]
              tunnel: w58 -> [w80]
              tunnel: [w69] -> w54
              stop <- w69 continue-if-true
              w79 = 0 ("lower limit")
              # "For each of the 8 Directions Check if a Roll and count. Stop when there is 4 or more"
              n22 = call "Pos_Get Direction.vim"("Direction"=w87) -> ("Position"=w85:T2)  [unwired: 10 in]
              n23 = Add(x=w86, y=w85) -> (x+y=w84:T2)
              n24 = Unbundle By Name(w84) -> ("R"=w83:i32, "C"=w82:i32)
              n25 = In Range and Coerce(upper limit=w80, x=w83, lower limit=w79) -> (coerced(x)=w74:i32, In Range?=w78:bool)
              n26 = In Range and Coerce(upper limit=w81, x=w82, lower limit=w79) -> (coerced(x)=w75:i32, In Range?=w77:bool)
              n27 = And(x=w78, y=w77) -> (x .and. y?=w76:bool)
              n28 = case shown="True" w76 {
                tunnel: w75 -> [_ w92]
                tunnel: w74 -> [_ w93]
                tunnel: w73 -> [_ w94]
                tunnel: w72 -> [w88 w90]
                tunnel: [w88 w89] -> w71
                frame False {
                  # "Out of Grid"
                }
                frame True {
                  # "Row and Column in Grid"
                  n29 = Index Array(array=w94, index (row)=w93, index (col)=w92) -> (element=w91:bool)
                  n30 = case shown="True" w91 {
                    tunnel: w90 -> [w95 w97]
                    tunnel: [w95 w96] -> w89
                    frame False {
                      # "No Ajacent Roll"
                    }
                    frame True {
                      # "Ajacent Roll Present"
                      n31 = Increment(x=w97) -> (x+1=w96:i32)
                    }
                  }
                }
              }
              n32 = Less?(x=w71, y=4) -> (x < y?=w69:bool)
            }
            n33 = case shown="True" w54 {
              tunnel: [w62 w65] -> w56
              tunnel: w55 -> [w62 w64]
              tunnel: w53 -> [_ w63]
              frame False {
                # "Roll to Keep"
              }
              frame True {
                # "Roll To Remove"
                n34 = Unbundle By Name(w63) -> ("R"=w68:i32, "C"=w67:i32)
                n35 = Replace Array Subset(array=w64, new element=FALSE ("new element/subarray"), index (row)=w68, index (col)=w67) -> (w65:bool[][])
              }
            }
          }
        }
      }
    }
    "Array" <- w24
    n36 = Boolean To (0,1)(Boolean=w28) -> (0, 1=w26:i16[])
    n37 = Or Array Elements(Boolean array=w28) -> (logical OR=w29:bool)
    n38 = To Unsigned Long Integer(number=w26) -> (unsigned 32bit integer=w27:u32[])
    n39 = Add Array Elements(numeric array=w27) -> (sum=w25:u32)
    "sum" <- w25
  }
  n40 = Add Array Elements(numeric array=w2) -> (sum=w1:u32)
  "Answer" <- w1
  n41 = Equal?(x=w4, y=w1) -> (x = y?=→"MATCH":bool)
